vi "SSL_enable_hostname_checks.vi"(8 "error in (no error)":errorcluster, 9 "Verification Flags":T1 items=["None"=0, "X509_CHECK_FLAG_ALWAYS_CHECK_SUBJECT"=1, "X509_CHECK_FLAG_NO_WILDCARDS"=2, "X509_CHECK_FLAG_NO_PARTIAL_WILDCARDS"=4, "X509_CHECK_FLAG_MULTI_LABEL_WILDCARDS"=8, "X509_CHECK_FLAG_SINGLE_LABEL_SUBDOMAINS"=16], 10 "Hostname":string, 11 "SSL in":refnum<class "SSL.lvclass">) -> (0 "error out":errorcluster, 3 "SSL out":refnum<class "SSL.lvclass">)   [LabVIEW 2013, in "OpenSSL Socket.lvlib" / "SSL.lvclass"]
uses:
  SSL.lvclass
  X509_Host_Verify_Flags.ctl
  SSL-Lib/SSL-Lib.lvclass/SSL-Lib.ctl
  SSL.lvclass/SSL.ctl
  SSL-Lib/Read Crypto Library Path.vi
  SSL-Lib/Read SSL Library Path.vi
  Read Handle.vi
  SSL-Lib/SSL-Lib.lvclass
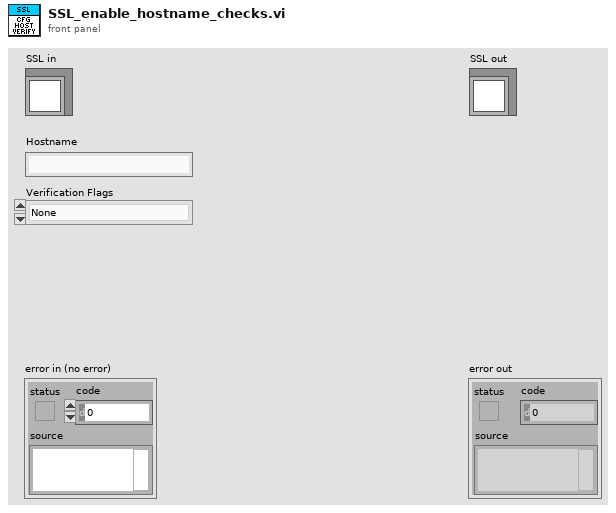
[diagram p1: front panel]
types:
  T1 = typedef "OpenSSL Socket.lvlib/SSL.lvclass/X509_Host_Verify_Flags.ctl" = u32
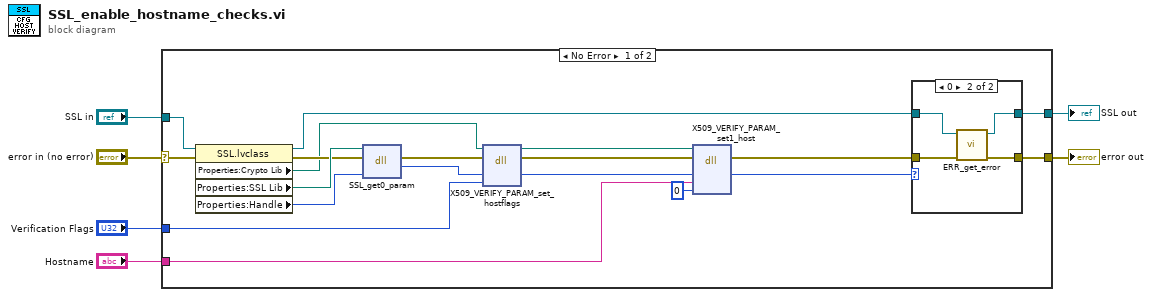
[diagram p0: block diagram]
diagram:
  n1 = case shown="No Error" "error in (no error)" {
    selector: "error in (no error)" -> [w24 w33]
    tunnel: [w8 w33] -> w5
    tunnel: [w11 w32] -> w3
    tunnel: "SSL in" -> [w25 w32]
    tunnel: "Verification Flags" -> [w18 _]
    tunnel: "Hostname" -> [w14 _]
    frame No Error {
      n2 = property class="SSL.lvclass"(reference=w25, error in=w24) -> (reference out=w10:refnum<class "SSL.lvclass">, error out=w21:errorcluster, "Properties:Crypto Lib"=w16:path, "Properties:SSL Lib"=w22:path, "Properties:Handle"=w23:u64)
      n3 = dll-call lib="C:/Program Files (x86)/National Instruments/Shared/nissl/NIssleay32.dll" fn="SSL_get0_param"(path in=w22, error in=w21, "SSL"=w23) -> (error out=w20:errorcluster, "param"=w19:u64)  [unwired: 2 in, 1 out]
      n4 = dll-call lib="C:/Program Files (x86)/National Instruments/Shared/nissl/NIlibeay32.dll" fn="X509_VERIFY_PARAM_set_hostflags"(path in=w16, error in=w20, "param"=w19, "flags"=w18) -> (path out=w15:path, error out=w12:errorcluster, "param"=w17:u64)  [unwired: 3 in]
      n5 = dll-call lib="C:/Program Files (x86)/National Instruments/Shared/nissl/NIlibeay32.dll" fn="X509_VERIFY_PARAM_set1_host"(path in=w15, error in=w12, "param"=w17, "name"=w14, "namelen"=u32 0) -> (error out=w13:errorcluster, "param"=w9:u64)  [unwired: 4 in, 1 out]
      n6 = case shown="0" w9 {
        tunnel: w13 -> [w26 w31]
        tunnel: [w27 w30] -> w11
        tunnel: w10 -> [w27 w29]
        tunnel: [w26 w28] -> w8
        frame Default {
        }
        frame 0 {
          n7 = call "ERR_get_error.vi"("error in (no error)"=w31, "SSL-Lib in"=w29) -> ("error out"=w28:errorcluster, "SSL-Lib out"=w30:refnum<class "SSL.lvclass">)  [unwired: 8 in]
        }
      }
    }
    frame Error {
    }
  }
  "error out" <- w5
  "SSL out" <- w3
